vi "TH_Utvärdering.vi"(6 "Medelvärdes-\nbildning":u16(ring) items=["Ingen", "Dynamisk", "6 timmar", "24 timmar"], 7 "Input Dates":T2={"Start År - 1"=0, "Start Månad - 1"=9, "Start Dag - 1"=1, "Slut År - 1"=0, "Slut Månad - 1"=9, "Slut Dag - 1"=1}) -> (1 "Min-X":dbl format="%.2f", 2 "Max-X":dbl format="%.2f", 3 "XY Graph":T1(graph))   [LabVIEW 2014]
uses:
  <vilib>/Analysis/baseanly.llb/Mean (DBL).vi
  <vilib>/Analysis/NI_AALBase.lvlib
panel:
  out "ArrayRows":dbl
  out "Array":dbl[][](array[numeric]) format="%.1f"
  out "Filesize":dbl
  out "Loading File....":path
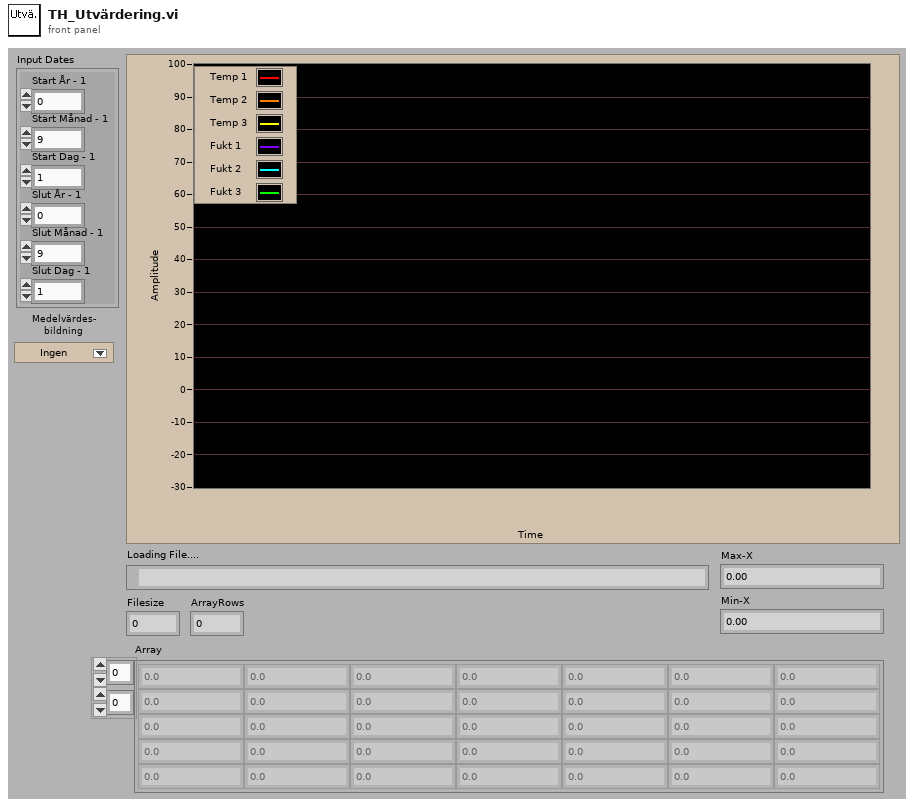
[diagram p1: front panel]
types:
  T1 = cluster{cluster{"Numeric":dbl, "Numeric":dbl}[]}[]
  T2 = cluster{"Start År - 1":u16, "Start Månad - 1":u16, "Start Dag - 1":u16, "Slut År - 1":u16, "Slut Månad - 1":u16, "Slut Dag - 1":u16}
  T3 = enum16{"open", "open or create", "create or replace", "create", "open (read only)"}
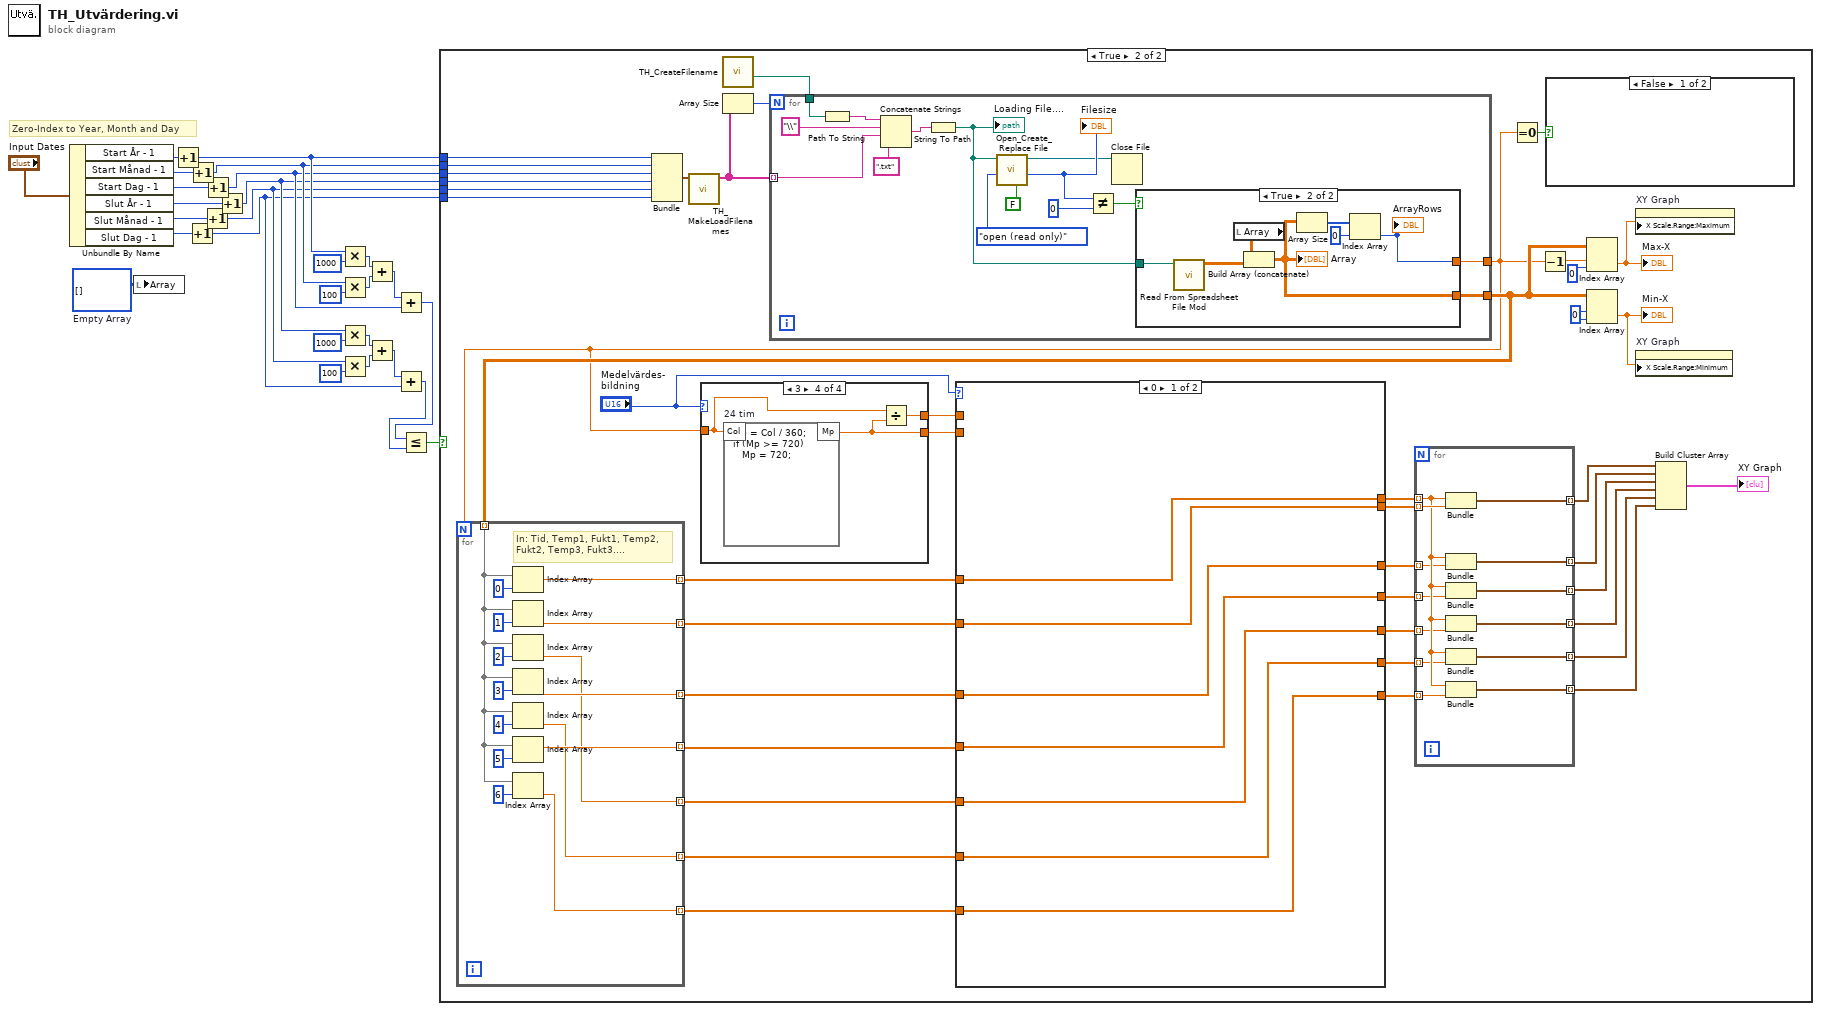
[diagram p0: block diagram]
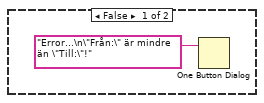
[diagram p2: hidden frame]
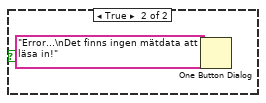
[diagram p3: hidden frame]
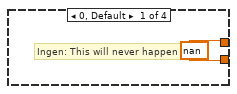
[diagram p4: hidden frame]
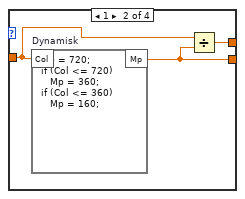
[diagram p5: hidden frame]
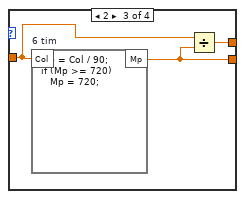
[diagram p6: hidden frame]
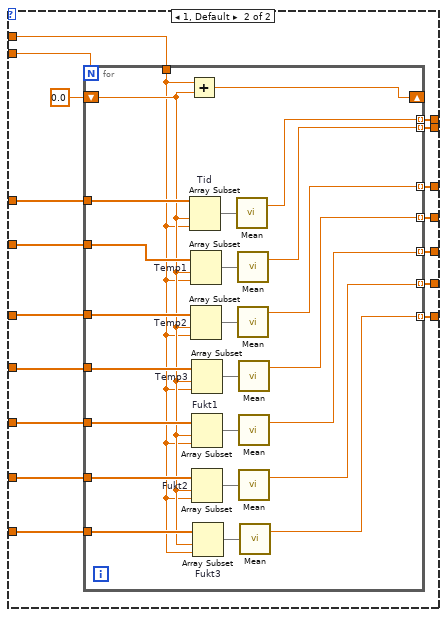
[diagram p7: hidden frame]
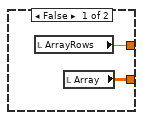
[diagram p8: hidden frame]
diagram:
  w20 = i32[][] []  # Empty Array
  # "Zero-Index to Year, Month and Day"
  n1 = Unbundle By Name("Input Dates") -> ("Start År - 1"=w26:u16, "Start Månad - 1"=w25:u16, "Start Dag - 1"=w24:u16, "Slut År - 1"=w23:u16, "Slut Månad - 1"=w22:u16, "Slut Dag - 1"=w21:u16)
  n2 = local write "Array"(w20) -> ()
  n3 = Increment(x=w26) -> (x+1=w18:u16)
  n4 = Increment(x=w21) -> (x+1=w4:u16)
  n5 = Increment(x=w25) -> (x+1=w16:u16)
  n6 = Increment(x=w22) -> (x+1=w5:u16)
  n7 = Increment(x=w24) -> (x+1=w13:u16)
  n8 = Increment(x=w23) -> (x+1=w6:u16)
  n9 = Multiply(x=w18, y=1000) -> (x*y=w15:i32)
  n10 = Multiply(x=w16, y=100) -> (x*y=w14:i32)
  n11 = Multiply(x=w6, y=1000) -> (x*y=w9:i32)
  n12 = Multiply(x=w5, y=100) -> (x*y=w10:i32)
  n13 = Add(x=w15, y=w14) -> (x+y=w12:i32)
  n14 = Add(x=w9, y=w10) -> (x+y=w11:i32)
  n15 = Add(x=w12, y=w13) -> (x+y=w2:i32)
  n16 = Add(x=w11, y=w4) -> (x+y=w1:i32)
  n17 = Less Or Equal?(x=w2, y=w1) -> (x <= y?=w3:bool)
  n18 = case shown="True" w3 {
    tunnel: w18 -> [_ w70]
    tunnel: w16 -> [_ w69]
    tunnel: w13 -> [_ w68]
    tunnel: w6 -> [_ w67]
    tunnel: w5 -> [_ w66]
    tunnel: w4 -> [_ w65]
    frame False {
      n19 = One Button Dialog(message="Error...\n\"Från:\" är mindre än \"Till:\"!") -> ()  [unwired: 1 in, 1 out]
    }
    frame True {
      w60 = 0 ("Index (row)")
      n20 = Bundle(w70, w69, w68, w67, w66, w65) -> (w64:cluster{u16, u16, u16, u16, u16, u16})  [unwired: 1 in]
      n21 = call "TH_MakeLoadFilenames.vi"("Input Dates"=w64) -> ("Filenames"=w62:string[])  [unwired: 6 in]
      n22 = call "TH_CreateFilename.vi"() -> ("DataPath"=w61:path)  [unwired: 5 in, 2 out]
      n23 = Array Size(array=w62) -> (size(s)=w63:i32)
      n24 = for {
        N: w63 -> [_]
        tunnel: w62 -> [w169] mode=indexing
        tunnel: w61 -> [w172]
        tunnel: [w159] -> w54
        tunnel: [w158] -> w29
        n25 = Path To String(path=w172) -> (string=w171:string)
        n26 = Concatenate Strings(w171, "\\", w169, ".txt") -> (w168:string)
        n27 = String To Path(string=w168) -> (path=w163:path)
        "Loading File...." <- w163
        n28 = call <vilib>:"Open_Create_Replace File.vi"("advisory dialog? (display:T)"=FALSE, "function (open:0)"=T3."open (read only)", "file path"=w163) -> ("file size (bytes)"=w165:i32, "refnum"=w161:refnum<file>)  [unwired: 5 in, 2 out]
        "Filesize" <- w165
        n29 = Not Equal?(x=w165, y=0) -> (x != y?=w166:bool)
        n30 = Close File(refnum=w161) -> ()  [unwired: 1 in, 2 out]
        n31 = case shown="True" w166 {
          tunnel: w163 -> [_ w181]
          tunnel: [w174 w176] -> w159
          tunnel: [w173 w175] -> w158
          frame False {
            n32 = local read "ArrayRows"() -> (w173:dbl)
            n33 = local read "Array"() -> (w174:dbl[][])
          }
          frame True {
            n34 = call "Read From Spreadsheet File Mod.vi"("file path (dialog if empty)"=w181) -> ("all rows"=w179:dbl[][])  [unwired: 6 in, 4 out]
            n35 = local read "Array"() -> (w180:dbl[][])
            n36 = Build Array (concatenate)(w180, w179) -> (w176:dbl[][])
            "Array" <- w176
            n37 = Array Size(array=w176) -> (size(s)=w178:i32[])
            n38 = Index Array(array=w178, index=0 ("Index")) -> (element=w175:i32)
            "ArrayRows" <- w175
          }
        }
      }
      n39 = for {
        N: w29 -> [_]
        tunnel: w54 -> [w150] mode=indexing
        tunnel: [w144] -> w53 mode=indexing
        tunnel: [w149] -> w52 mode=indexing
        tunnel: [w148] -> w51 mode=indexing
        tunnel: [w147] -> w50 mode=indexing
        tunnel: [w146] -> w49 mode=indexing
        tunnel: [w145] -> w48 mode=indexing
        tunnel: [w143] -> w47 mode=indexing
        # "In: Tid, Temp1, Fukt1, Temp2,\nFukt2, Temp3, Fukt3...."
        n40 = Index Array(array=w150, index=0 ("Index")) -> (element=w144:dbl)
        n41 = Index Array(array=w150, index=1 ("Index")) -> (element=w149:dbl)
        n42 = Index Array(array=w150, index=2 ("Index")) -> (element=w146:dbl)
        n43 = Index Array(array=w150, index=3 ("Index")) -> (element=w148:dbl)
        n44 = Index Array(array=w150, index=4 ("Index")) -> (element=w145:dbl)
        n45 = Index Array(array=w150, index=5 ("Index")) -> (element=w147:dbl)
        n46 = Index Array(array=w150, index=6 ("Index")) -> (element=w143:dbl)
      }
      n47 = case shown="3" "Medelvärdes-\nbildning" {
        tunnel: [w72 w74 w77 w80] -> w33
        tunnel: w29 -> [_ w73 w76 w79]
        tunnel: [w72 w75 w78 w81] -> w32
        frame 0, Default {
          w72 = nan
          # "Ingen: This will never happen"
        }
        frame 1 {
          n48 = formula code="Mp = 720;\nif (Col <= 720)\n   Mp = 360;\nif (Col <= 360)\n   Mp = 160;" "Dynamisk"("Col"=w73) -> ("Mp"=w74:dbl)
          n49 = Divide(x=w73, y=w74) -> (x/y=w75:dbl)
        }
        frame 2 {
          n50 = formula code="Mp = Col / 90;\nif (Mp >= 720)\n   Mp = 720;" "6 tim"("Col"=w76) -> ("Mp"=w77:dbl)
          n51 = Divide(x=w76, y=w77) -> (x/y=w78:dbl)
        }
        frame 3 {
          n52 = formula code="Mp = Col / 360;\nif (Mp >= 720)\n   Mp = 720;" "24 tim"("Col"=w79) -> ("Mp"=w80:dbl)
          n53 = Divide(x=w79, y=w80) -> (x/y=w81:dbl)
        }
      }
      n54 = case shown="0" "Medelvärdes-\nbildning" {
        tunnel: w33 -> [_ w90]
        tunnel: w53 -> [w88 w105]
        tunnel: w52 -> [w87 w104]
        tunnel: w51 -> [w86 w101]
        tunnel: w50 -> [w85 w99]
        tunnel: w49 -> [w84 w98]
        tunnel: w48 -> [w83 w96]
        tunnel: w47 -> [w82 w97]
        tunnel: [w88 w102] -> w46
        tunnel: [w87 w100] -> w45
        tunnel: [w86 w95] -> w44
        tunnel: [w85 w94] -> w43
        tunnel: [w84 w93] -> w42
        tunnel: [w83 w92] -> w41
        tunnel: [w82 w91] -> w40
        tunnel: w32 -> [_ w89]
        frame 0 {
        }
        frame 1, Default {
          n55 = for {
            N: w90 -> [_]
            tunnel: w89 -> [w106]
            tunnel: w105 -> [w129]
            tunnel: w104 -> [w116]
            shift-right: [w128] -> _
            shift-left: 0.0 -> [w107]
            tunnel: [w126] -> w102 mode=indexing
            tunnel: w101 -> [w115]
            tunnel: w99 -> [w114]
            tunnel: w98 -> [w113]
            tunnel: [w122] -> w100 mode=indexing
            tunnel: w96 -> [w118]
            tunnel: w97 -> [w117]
            tunnel: [w112] -> w95 mode=indexing
            tunnel: [w111] -> w94 mode=indexing
            tunnel: [w110] -> w93 mode=indexing
            tunnel: [w109] -> w92 mode=indexing
            tunnel: [w108] -> w91 mode=indexing
            n56 = Add(x=w106, y=w107) -> (x+y=w128:dbl)
            n57 = Array Subset "Tid"(array=w129, index=w107, length=w106) -> (w127:dbl[])
            n58 = Array Subset "Temp1"(array=w116, index=w107, length=w106) -> (w125:dbl[])
            n59 = Array Subset "Temp2"(array=w115, index=w107, length=w106) -> (w124:dbl[])
            n60 = Array Subset "Temp3"(array=w114, index=w107, length=w106) -> (w123:dbl[])
            n61 = Array Subset "Fukt1"(array=w113, index=w107, length=w106) -> (w119:dbl[])
            n62 = Array Subset "Fukt2"(array=w118, index=w107, length=w106) -> (w120:dbl[])
            n63 = Array Subset "Fukt3"(array=w117, index=w107, length=w106) -> (w121:dbl[])
            n64 = call-poly <vilib>:"Mean.vi"("X"=w127) -> ("mean"=w126:dbl)  [unwired: 1 out]
            n65 = call-poly <vilib>:"Mean.vi"("X"=w125) -> ("mean"=w122:dbl)  [unwired: 1 out]
            n66 = call-poly <vilib>:"Mean.vi"("X"=w124) -> ("mean"=w112:dbl)  [unwired: 1 out]
            n67 = call-poly <vilib>:"Mean.vi"("X"=w123) -> ("mean"=w111:dbl)  [unwired: 1 out]
            n68 = call-poly <vilib>:"Mean.vi"("X"=w119) -> ("mean"=w110:dbl)  [unwired: 1 out]
            n69 = call-poly <vilib>:"Mean.vi"("X"=w120) -> ("mean"=w109:dbl)  [unwired: 1 out]
            n70 = call-poly <vilib>:"Mean.vi"("X"=w121) -> ("mean"=w108:dbl)  [unwired: 1 out]
          }
        }
      }
      n71 = for {
        tunnel: [w142] -> w39 mode=indexing
        tunnel: [w137] -> w38 mode=indexing
        tunnel: [w141] -> w37 mode=indexing
        tunnel: [w140] -> w36 mode=indexing
        tunnel: [w139] -> w35 mode=indexing
        tunnel: [w138] -> w34 mode=indexing
        tunnel: w46 -> [w135] mode=indexing
        tunnel: w45 -> [w136] mode=indexing
        tunnel: w44 -> [w134] mode=indexing
        tunnel: w43 -> [w133] mode=indexing
        tunnel: w42 -> [w132] mode=indexing
        tunnel: w41 -> [w131] mode=indexing
        tunnel: w40 -> [w130] mode=indexing
        n72 = Bundle("mean"=w135, "mean"=w136) -> (w142:cluster{"mean":dbl, "mean":dbl})  [unwired: 1 in]
        n73 = Bundle("mean"=w135, "mean"=w134) -> (w137:cluster{"mean":dbl, "mean":dbl})  [unwired: 1 in]
        n74 = Bundle("mean"=w135, "mean"=w133) -> (w141:cluster{"mean":dbl, "mean":dbl})  [unwired: 1 in]
        n75 = Bundle("mean"=w135, "mean"=w132) -> (w140:cluster{"mean":dbl, "mean":dbl})  [unwired: 1 in]
        n76 = Bundle("mean"=w135, "mean"=w131) -> (w139:cluster{"mean":dbl, "mean":dbl})  [unwired: 1 in]
        n77 = Bundle("mean"=w135, "mean"=w130) -> (w138:cluster{"mean":dbl, "mean":dbl})  [unwired: 1 in]
      }
      n78 = Equal To 0?(x=w29) -> (x = 0?=w30:bool)
      n79 = Decrement(x=w29) -> (x-1=w58:dbl)
      n80 = case shown="False" w30 {
        frame False {
        }
        frame True {
          n81 = One Button Dialog(message="Error...\nDet finns ingen mätdata att läsa in!") -> ()  [unwired: 1 in, 1 out]
        }
      }
      n82 = Index Array(array=w54, index (row)=w58, index (col)=0 ("Disabled Index (col)")) -> (element=w55:dbl)
      "Max-X" <- w55
      n83 = Index Array(array=w54, index (row)=w60, index (col)=w60) -> (element=w56:dbl)
      "Min-X" <- w56
      n84 = property on="XY Graph" class="XYGraph (strict)"("X Scale.Range:Maximum"=w55) -> ()  [unwired: 2 in, 2 out]
      n85 = property on="XY Graph" class="XYGraph (strict)"("X Scale.Range:Minimum"=w56) -> ()  [unwired: 2 in, 2 out]
      n86 = Build Cluster Array(w39, w38, w37, w36, w35, w34) -> (→"XY Graph":cluster{cluster{"mean":dbl, "mean":dbl}[]}[])
    }
  }
